vi "Core_Connect.vi"(8 "error in (no error)":errorcluster, 11 "HSMS Class in":refnum<class "HSMS Class.lvclass">) -> (0 "error out":errorcluster, 3 "HSMS Class out":refnum<class "HSMS Class.lvclass">)   [LabVIEW 2020, in "SECS Communication.lvlib" / "HSMS Class.lvclass"]
uses:
  HSMS Class.lvclass
  HSMS Class.lvclass/HSMS Class.ctl
  Read Listener Refnum.vi
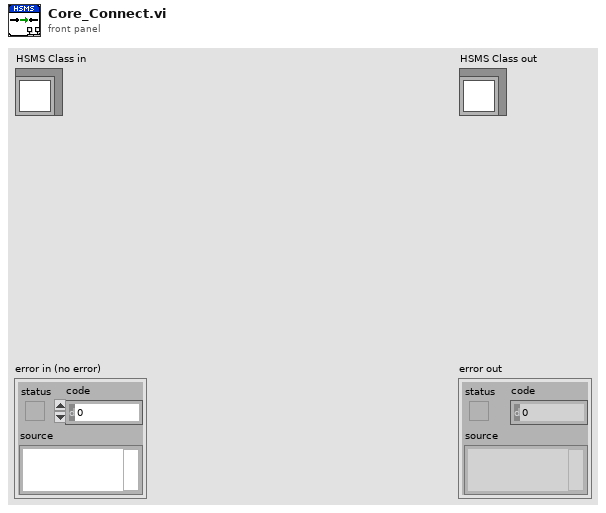
[diagram p1: front panel]
types:
  T1 = typedef "SECS Communication.lvlib/HSMS Class.lvclass/Role.ctl" = enum16{"Passive", "Active"}
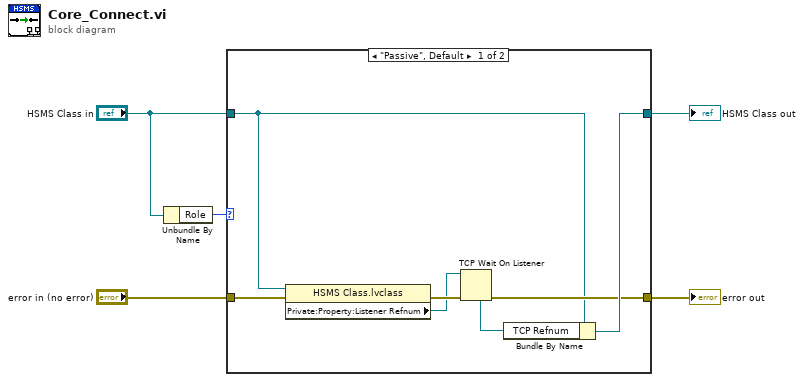
[diagram p0: block diagram]
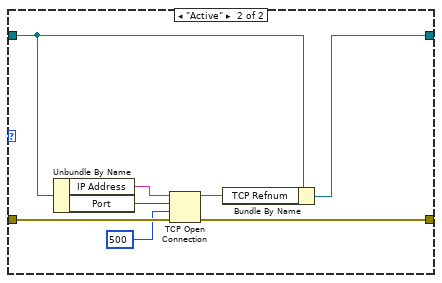
[diagram p2: hidden frame]
diagram:
  n1 = Unbundle By Name("HSMS Class in") -> ("Role"=w5:T1)
  n2 = case shown="\"Passive\", Default" w5 {
    tunnel: "HSMS Class in" -> [w8 w16]
    tunnel: "error in (no error)" -> [w9 w20]
    tunnel: [w10 w14] -> w2
    tunnel: [w11 w13] -> w1
    frame "Passive", Default {
      n3 = property class="HSMS Class.lvclass"(reference=w8, error in=w9) -> (error out=w7:errorcluster, "Private:Property:Listener Refnum"=w6:refnum<k5>)  [unwired: 1 out]
      n4 = TCP Wait On Listener(8:w7, 11:w6) -> (0:w10:errorcluster, 4:w12:refnum<k5>)  [unwired: 2 in, 3 out]
      n5 = Bundle By Name(cluster=w8, "TCP Refnum"=w12) -> (w11:refnum<class "HSMS Class.lvclass">)
    }
    frame "Active" {
      n6 = Unbundle By Name(w16) -> ("IP Address"=w18:string, "Port"=w19:u16)
      n7 = TCP Open Connection(address=w18, remote port or service name=w19, timeout ms (60000)=500, error in (no error)=w20) -> (connection ID=w15:refnum<k5>, error out=w14:errorcluster)  [unwired: 1 in]
      n8 = Bundle By Name(cluster=w16, "TCP Refnum"=w15) -> (w13:refnum<class "HSMS Class.lvclass">)
    }
  }
  "error out" <- w2
  "HSMS Class out" <- w1
